vi "22_1.vi"() -> ()   [LabVIEW 2020]
panel:
  out "sum":i32=33694
  in  "Switch":bool
  in  "Input":string="Player 1:\n28\n13\n25\n16\n38\n3\n14\n6\n29\n2\n47\n20\n35\n43\n30\n39\n21\n42\n50\n48\n23\n11\n34\n24\n41\n\nPlayer 2:\n27\n37\n9\n10\n17\n31\n19\n33\n40\n12\n32\n1\n18\n36\n49\n46\n26\n4\n45\n8\n15\n5\n44\n22\n7"
  in  "Input Test":string="Player 1:\n9\n2\n6\n3\n1\n\nPlayer 2:\n5\n8\n4\n7\n10"
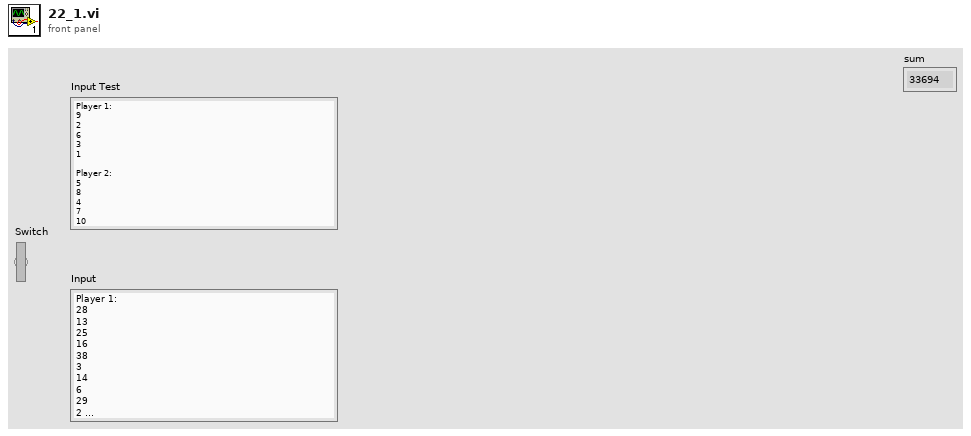
[diagram p1: front panel]
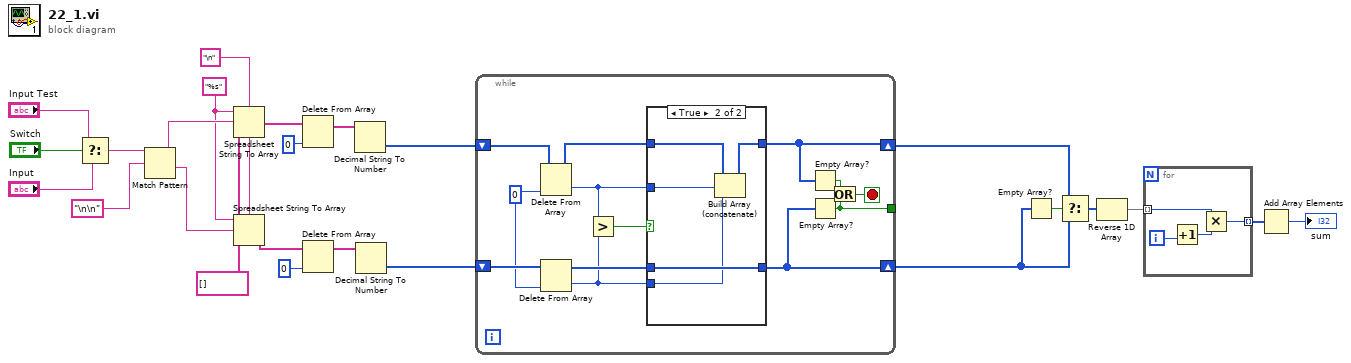
[diagram p0: block diagram]
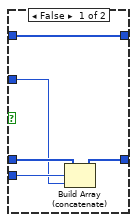
[diagram p2: hidden frame]
diagram:
  w19 = string[] []
  w16 = "\n"
  w18 = "%s"
  n1 = Select(t="Input Test", s="Switch", f="Input") -> (s? t:f=w22:string)
  n2 = Match Pattern(string=w22, regular expression="\n\n") -> (before substring=w20:string, after substring=w17:string)  [unwired: 1 in, 2 out]
  n3 = Spreadsheet String To Array(delimiter (Tab)=w16, format string=w18, spreadsheet string=w20, array type (2D Dbl)=w19) -> (array=w15:string[])
  n4 = Spreadsheet String To Array(delimiter (Tab)=w16, format string=w18, spreadsheet string=w17, array type (2D Dbl)=w19) -> (array=w14:string[])
  n5 = Delete From Array(array=w15, index=0) -> (array with subset deleted=w12:string[])  [unwired: 1 in, 1 out]
  n6 = Delete From Array(array=w14, index=0) -> (array with subset deleted=w11:string[])  [unwired: 1 in, 1 out]
  n7 = Decimal String To Number(string=w12) -> (number=w10:i32[])  [unwired: 2 in, 1 out]
  n8 = Decimal String To Number(string=w11) -> (number=w9:i32[])  [unwired: 2 in, 1 out]
  n9 = while {
    shift-right: [w29] -> w3
    shift-left: w10 -> [w35]
    shift-right: [w28] -> w1
    shift-left: w9 -> [w34]
    tunnel: [w36] -> _
    stop <- w38 stop-if-true
    w33 = 0
    n10 = Delete From Array(array=w35, index=w33) -> (deleted portion=w27:i32, array with subset deleted=w31:i32[])  [unwired: 1 in]
    n11 = Delete From Array(array=w34, index=w33) -> (deleted portion=w26:i32, array with subset deleted=w30:i32[])  [unwired: 1 in]
    n12 = Greater?(x=w27, y=w26) -> (0:w32:bool)
    n13 = case shown="True" w32 {
      tunnel: w31 -> [w43 w45]
      tunnel: [w43 w44] -> w29
      tunnel: [w39 w48] -> w28
      tunnel: w30 -> [w42 w48]
      tunnel: w27 -> [w40 w47]
      tunnel: w26 -> [w41 w46]
      frame False {
        n14 = Build Array (concatenate)(w42, w41, w40) -> (w39:i32[])
      }
      frame True {
        n15 = Build Array (concatenate)(w45, w47, w46) -> (w44:i32[])
      }
    }
    n16 = Empty Array?(array=w29) -> (empty?=w37:bool)
    n17 = Empty Array?(array=w28) -> (empty?=w36:bool)
    n18 = Or(x=w37, y=w36) -> (x .or. y?=w38:bool)
  }
  n19 = Empty Array?(array=w1) -> (empty?=w2:bool)
  n20 = Select(t=w3, s=w2, f=w1) -> (s? t:f=w8:i32[])
  n21 = Reverse 1D Array(array=w8) -> (reversed array=w7:i32[])
  n22 = for {
    tunnel: w7 -> [w50] mode=indexing
    tunnel: [w49] -> w6 mode=indexing
    i -> [w52]
    n23 = Increment(x=w52) -> (x+1=w51:i32)
    n24 = Multiply(x=w50, y=w51) -> (x*y=w49:i32)
  }
  n25 = Add Array Elements(numeric array=w6) -> (sum=→"sum":i32)
